vi "Write-to-file-by-value.vi"(8 "error in (no error)":errorcluster, 10 "Values to save":T1, 11 "SettingsFile in":refnum<class "SettingsFile.lvclass">) -> (0 "error out":errorcluster, 3 "SettingsFile out":refnum<class "SettingsFile.lvclass">)   [LabVIEW 2013, in "SettingsFile.lvlib" / "SettingsFile.lvclass"]
uses:
  SettingsFile.lvclass
  Values-to-save.ctl
  SettingsFile.lvclass/SettingsFile.ctl
  Errors.ctl
  <vilib>/Utility/xml.llb/Write to XML File(string).vi
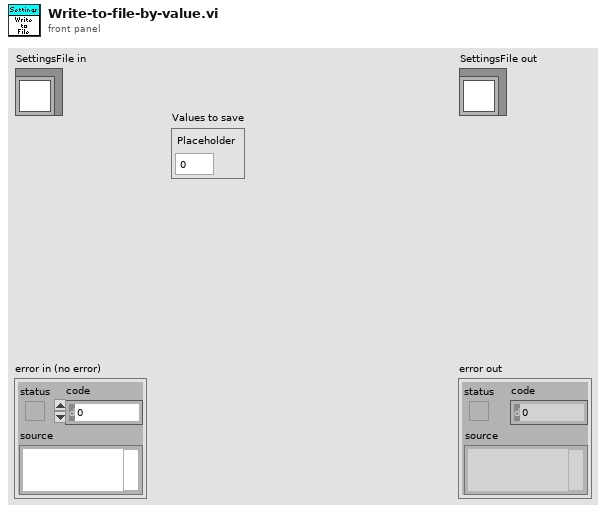
[diagram p1: front panel]
types:
  T1 = typedef "SettingsFile.lvlib/SettingsFile.lvclass/Values-to-save.ctl" = cluster{"Placeholder":dbl}
  T2 = typedef "SettingsFile.lvlib/SettingsFile.lvclass/Errors.ctl" = enum16{"Not implemented", "Command not recognized", "Invalid input", "No connection", "Timeout", "Invalid file type", "No file access"}
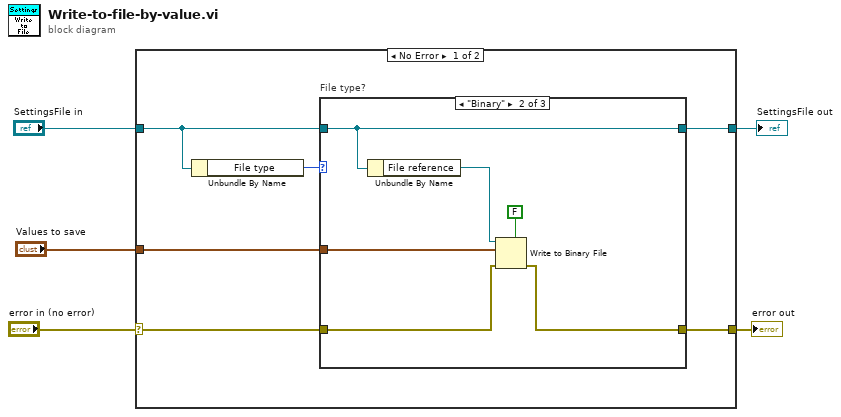
[diagram p0: block diagram]
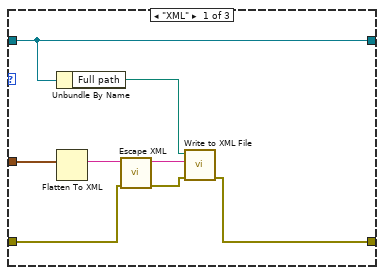
[diagram p2: hidden frame]
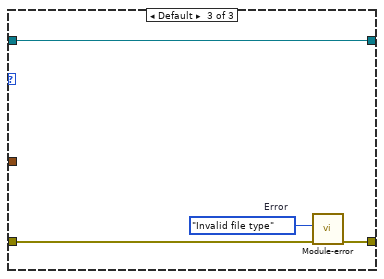
[diagram p3: hidden frame]
diagram:
  n1 = case shown="No Error" "error in (no error)" {
    selector: "error in (no error)" -> [w8 w31]
    tunnel: [w7 w31] -> w4
    tunnel: [w9 w30] -> w2
    tunnel: "SettingsFile in" -> [w10 w30]
    tunnel: "Values to save" -> [w6 _]
    frame No Error {
      n2 = Unbundle By Name(w10) -> ("File type"=w11:enum16{"XML", "INI", "Binary"})
      n3 = case "File type?" shown="\"Binary\"" w11 {
        tunnel: w10 -> [w14 w25 w29]
        tunnel: [w14 w25 w29] -> w9
        tunnel: w8 -> [w13 w22 w27]
        tunnel: [w12 w21 w28] -> w7
        tunnel: w6 -> [w16 w23 _]
        frame "XML" {
          n4 = Unbundle By Name(w14) -> ("Full path"=w15:path)
          n5 = Flatten To XML(anything=w16) -> (xml string=w18:string)
          n6 = call <vilib>:"Escape XML.vi"("error in (no error)"=w13, "XML String In"=w18) -> ("error out"=w17:errorcluster, "XML String Out"=w19:string)  [unwired: 8 in]
          n7 = call-poly <vilib>:"Write to XML File.vi"("error in (no error)"=w17, "XML Input"=w19, "XML File Path"=w15) -> ("error out"=w12:errorcluster)  [unwired: 6 in, 2 out]
        }
        frame "Binary" {
          n8 = Unbundle By Name(w25) -> ("File reference"=w24:refnum<file>)
          n9 = Write to Binary File(file (use dialog)=w24, data=w23, error in=w22, 5:FALSE) -> (error out=w21:errorcluster)  [unwired: 2 in, 2 out]
        }
        frame Default {
          w26 = Errors."Invalid file type"  # Error
          n10 = call "Module-error.vi"("error in (no error)"=w27, "Error"=w26) -> ("error out"=w28:errorcluster)  [unwired: 9 in]
        }
      }
    }
    frame Error {
    }
  }
  "error out" <- w4
  "SettingsFile out" <- w2
